vi "Get Paths.vi"(7 "Extension(txt)":string="txt", 8 "error in":errorcluster, 10 "VI name":string) -> (0 "error out":errorcluster, 2 "recived path":path, 3 "approved path":path)   [LabVIEW 2020, in "Approval Tests.lvlib"]
doc: "Generates 2 absolute paths based on the name of the calling unit test.\n\nname_of_unit_test.approved\nname_of_unit_test.actual"
uses:
  Approval Tests.lvlib
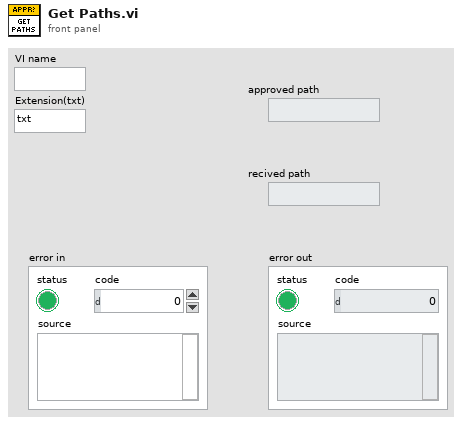
[diagram p1: front panel]
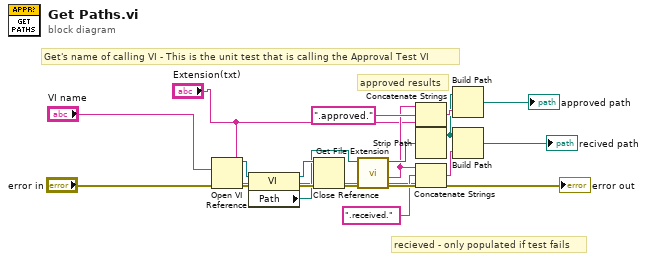
[diagram p0: block diagram]
diagram:
  # "recieved - only populated if test fails"
  # "approved results"
  # "Get's name of calling VI - This is the unit test that is calling the Approval Test VI"
  n1 = Open VI Reference(vi path="VI name", error in (no error)="error in") -> (vi reference=w11:refnum<vi>, error out=w15:errorcluster)  [unwired: 4 in]
  n2 = property on="Property Node" class="VI"(reference=w11, error in=w15) -> (reference out=w13:refnum<vi>, error out=w16:errorcluster, "Path"=w12:path)
  n3 = Close Reference(reference=w13, error in (no error)=w16) -> (error out=w17:errorcluster)
  n4 = call <vilib>:"Get File Extension.vi"("error in (no error)"=w17, "file"=w12) -> ("error out"=→"error out":errorcluster, "filename without extension"=w3:string, "dup file"=w8:path)  [unwired: 5 in, 2 out]
  n5 = Concatenate Strings(w3, ".approved." ("string"), "Extension(txt)") -> (w10:string)
  n6 = Strip Path(path=w8) -> (stripped path=w5:path)  [unwired: 1 out]
  n7 = Concatenate Strings(w3, ".received." ("string"), "Extension(txt)") -> (w6:string)
  n8 = Build Path(base path=w5, name or relative path=w10) -> (appended path=→"approved path":path)
  n9 = Build Path(base path=w5, name or relative path=w6) -> (appended path=→"recived path":path)
